vi "Send Default TV.vi"(8 "error in (no error)":errorcluster, 11 "Model in":refnum<class "Model.lvclass">) -> (0 "error out":errorcluster, 3 "Model out":refnum<class "Model.lvclass">)   [LabVIEW 2015, in "Model.lvclass"]
uses:
  Model.lvclass
  Model.lvclass/Model.ctl
  DAQmx/DAQmx.lvclass
  Calculators/Percentage To Turbo Valve Voltage/Percentage To Turbo Valve Voltage.lvclass
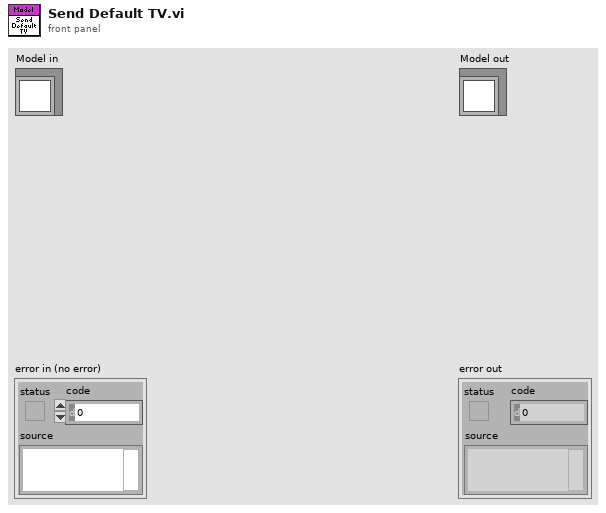
[diagram p1: front panel]
types:
  T1 = typedef "FAMT Typedefs.lvlib/Turbo Valve Settings.ctl" = cluster{"Bias":u16, "Minimum Voltage":dbl, "Maximum Voltage":dbl, "Off Value":dbl}
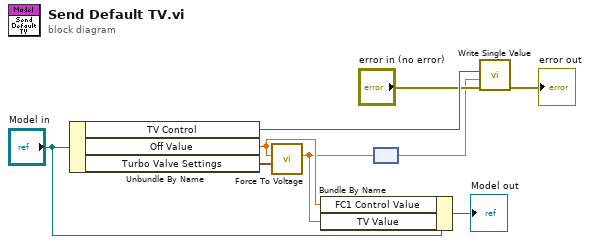
[diagram p0: block diagram]
diagram:
  n1 = Unbundle By Name("Model in") -> ("TV Control"=w9:refnum<k21>, "Off Value"=w3:dbl, "Turbo Valve Settings"=w5:T1)
  n2 = call "Force To Voltage.vi"("Turbo Valve Settings"=w5, "Percentage"=w3) -> ("Voltage"=w2:dbl[unit])  [unwired: 7 in, 2 out]
  n3 = Bundle By Name(cluster="Model in", "FC1 Control Value"=w3, "TV Value"=w2) -> (→"Model out":refnum<class "Model.lvclass">)
  n4 = node(w2) -> (w4:dbl)
  n5 = call "Write Single Value.vi"("error in (no error)"="error in (no error)", "Value"=w4, "Channel"=w9) -> ("error out"=→"error out":errorcluster)  [unwired: 7 in, 1 out]
